vi "IntakeForTime.vi"() -> ()   [LabVIEW 2017]
uses:
  Framework/Robot Global Data.vi
panel:
  in  "Time":dbl
  in  "Speed":dbl
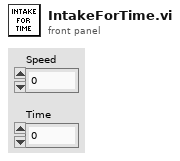
[diagram p1: front panel]
types:
  T1 = typedef "Command Status Info.ctl" = cluster{"Name":string, "Status":T2, "notifier out":T3}
  T2 = typedef "Completion Status.ctl" = enum16{"Successful", "Aborted", "Incomplete"}
  T3 = typedef "Completion Notifier.ctl" = refnum<notifier>
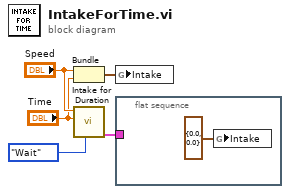
[diagram p0: block diagram]
diagram:
  n1 = Bundle("Speed"="Speed", "Time"="Time") -> (w5:cluster{"Speed":dbl, "Time":dbl})  [unwired: 1 in]
  n2 = call "Intake for Duration.vi"("Synchronization"=enum16{"Start", "Wait"}."Wait", "Duration (s)"="Time", "Speed"="Speed") -> ("Command Info Out"=w2:T1)  [unwired: 8 in]
  n3 = global write "Robot Global Data.vi" "Intake"(w5) -> ()
  n4 = flat-sequence {
    tunnel: w2 -> [_]
    frame #0 {
      n5 = global write "Robot Global Data.vi" "Intake"(cluster{"Drive Speed":dbl, "Drive Time":dbl} {"Drive Speed"=0.0, "Drive Time"=0.0} ("Drive")) -> ()
    }
  }
